vi "SendStreamCommand.vi"(8 "error in (no error)":errorcluster, 11 "Nav6DevRef":T1) -> (0 "error out":errorcluster, 3 "Nav6DevRef":T1)   [LabVIEW 2014, in "Nav6.lvlib"]
uses:
  Nav6.lvlib
  Nav6DevRef.ctl
  <vilib>/Rock Robotics/WPI/SerialPort/WPI_SerialPortRef.ctl
  Nav6Mode.ctl
panel:
  out "StreamCommand":string
  out "UpdateRate":u8
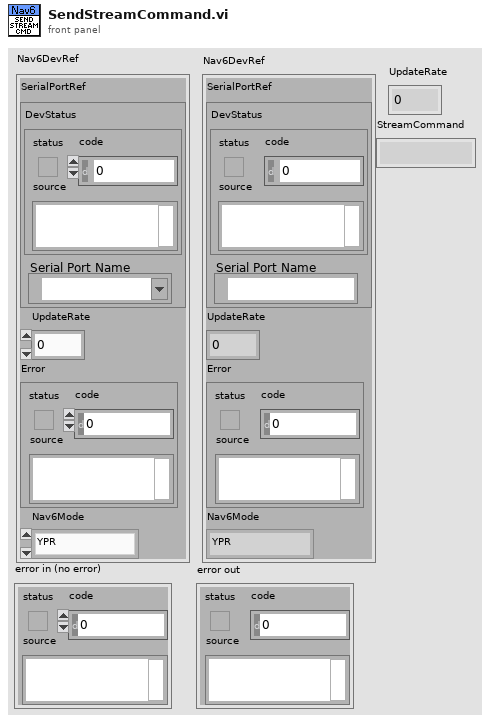
[diagram p1: front panel]
types:
  T1 = typedef "Nav6.lvlib/Nav6DevRef.ctl" = cluster{"SerialPortRef":T2, "UpdateRate":u8, "Error":errorcluster, "Nav6Mode":T3}
  T2 = typedef "WPI_SerialPortRef.ctl" = cluster{"DevStatus":errorcluster, "Serial Port Name":refnum<visa-resource-name>}
  T3 = typedef "Nav6.lvlib/Nav6Mode.ctl" = enum16{"YPR", "Gyro", "Quaternion"}
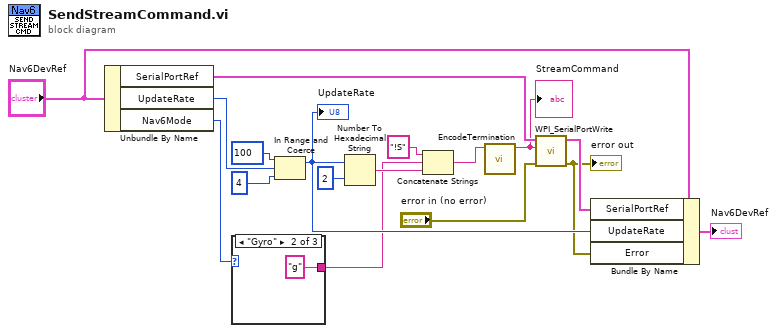
[diagram p0: block diagram]
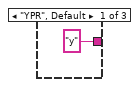
[diagram p2: hidden frame]
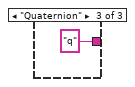
[diagram p3: hidden frame]
diagram:
  n1 = Unbundle By Name("Nav6DevRef") -> ("SerialPortRef"=w12:T2, "UpdateRate"=w13:u8, "Nav6Mode"=w2:T3)
  n2 = case shown="\"Gyro\"" w2 {
    tunnel: ["y" "g" "q"] -> w1
    frame "YPR", Default {
    }
    frame "Gyro" {
    }
    frame "Quaternion" {
    }
  }
  n3 = In Range and Coerce(upper limit=u8 100, x=w13, lower limit=u8 4) -> (coerced(x)=w5:u8)  [unwired: 1 out]
  "UpdateRate" <- w5
  n4 = Number To Hexadecimal String(1:i16 2 ("width (-)"), 2:w5) -> (0:w9:string)
  n5 = Concatenate Strings("!S" ("string"), w1, w9) -> (w17:string)
  n6 = call "EncodeTermination.vi"("String in"=w17) -> ("String out"=w11:string)  [unwired: 10 in]
  "StreamCommand" <- w11
  n7 = call <vilib>:"WPI_SerialPortWrite.vi"("error in (no error)"="error in (no error)", "Buffer"=w11, "SerialPortRef"=w12) -> ("error out"=w4:errorcluster, "SerialPortRef"=w6:T2)  [unwired: 6 in, 1 out]
  "error out" <- w4
  n8 = Bundle By Name(cluster="Nav6DevRef", "SerialPortRef"=w6, "UpdateRate"=w5, "Error"=w4) -> (→"Nav6DevRef":T1)
